vi "RM.initDatabase.vi"(8 "error in":errorcluster) -> (0 "error out":errorcluster, 3 "reservation DB out":variant)   [LabVIEW 2016, in "FPGA Addon Shared.lvlib"]
uses:
  FPGA Addon Shared.lvlib
  RM.resourceDirection.ctl
  RM.resourceType.ctl
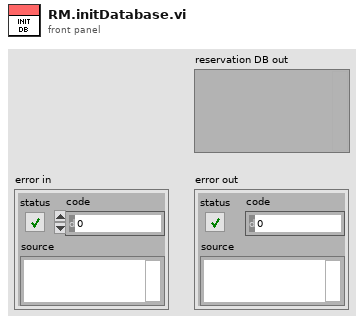
[diagram p1: front panel]
types:
  T1 = typedef "FPGA Addon Shared.lvlib/RM.resourceType.ctl" = enum16{"Scalar", "Waveform"}
  T2 = typedef "FPGA Addon Shared.lvlib/RM.resourceDirection.ctl" = enum16{"To FPGA", "From FPGA"}
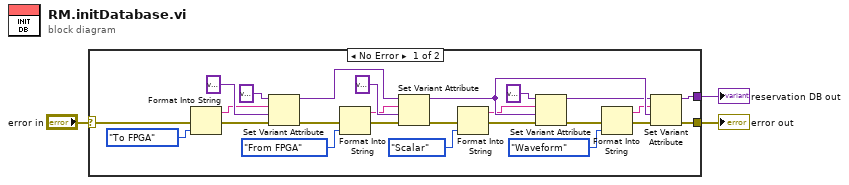
[diagram p0: block diagram]
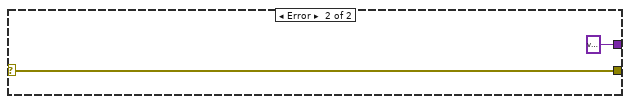
[diagram p2: hidden frame]
diagram:
  n1 = case shown="No Error" "error in" {
    selector: "error in" -> [w11 w29]
    tunnel: [w23 variant] -> w3
    tunnel: [w22 w29] -> w2
    frame No Error {
      n2 = Format Into String(error in=w11, RM.resourceDirection."To FPGA" ("Direction")) -> (resulting string=w17:string, error out=w10:errorcluster)  [unwired: 2 in]
      n3 = Set Variant Attribute(Variant=variant, name=w17, value=variant, error in=w10) -> (Variant out=w26:variant, error out=w9:errorcluster)  [unwired: 1 out]
      n4 = Format Into String(error in=w9, RM.resourceDirection."From FPGA" ("Direction")) -> (resulting string=w16:string, error out=w8:errorcluster)  [unwired: 2 in]
      n5 = Set Variant Attribute(Variant=w26, name=w16, value=variant, error in=w8) -> (Variant out=w25:variant, error out=w7:errorcluster)  [unwired: 1 out]
      n6 = Format Into String(error in=w7, RM.resourceType."Scalar" ("Resource Type")) -> (resulting string=w13:string, error out=w6:errorcluster)  [unwired: 2 in]
      n7 = Set Variant Attribute(Variant=variant, name=w13, value=w25, error in=w6) -> (Variant out=w24:variant, error out=w5:errorcluster)  [unwired: 1 out]
      n8 = Format Into String(error in=w5, RM.resourceType."Waveform" ("Resource Type")) -> (resulting string=w12:string, error out=w4:errorcluster)  [unwired: 2 in]
      n9 = Set Variant Attribute(Variant=w24, name=w12, value=w25, error in=w4) -> (Variant out=w23:variant, error out=w22:errorcluster)  [unwired: 1 out]
    }
    frame Error {
    }
  }
  "reservation DB out" <- w3
  "error out" <- w2
